vi "runStraight1Tote.vi"(11 "Distance In":dbl) -> ()   [LabVIEW 2015]
uses:
  Robot Global Data.vi
  <vilib>/addons/control/pid/NI_PID_pid.lvlib
  <vilib>/addons/control/pid/pid.llb/PID (DBL).vi
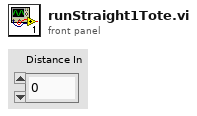
[diagram p1: front panel]
types:
  T1 = typedef "WPI_GyroDevRef.ctl" = cluster{"DevStatus":errorcluster, "Analog Channel":T2, "Offset":dbl, "Gain (VoltsPerDegree/Second)":dbl, "Gyro Type":enum16{"Analog", "XRS450"}, "Handle":i32, "SPI Bus":T3, "Device Found":bool, "Sample Rate":dbl, "Calibrate On Open":bool}
  T2 = typedef "FPGA_AIChannel.ctl" = enum8{"AI 0", "AI 1", "AI 2", "AI 3", "AI MXP 0", "AI MXP 1", "AI MXP 2", "AI MXP 3", "Invalid"}
  T3 = typedef "spi_bus.ctl" = enum16{"SPI On-Board, CS0", "SPI On-Board, CS1", "SPI On-Board, CS2", "SPI On-Board, CS3", "SPI MXP", "Invalid"}
  T4 = typedef "WPI_EncoderDevRef.ctl" = cluster{"DevStatus":errorcluster, "EncoderIndex":T5, "CounterIndex":T6, "DistancePerCount":dbl, "Decoding Type":T7}
  T5 = typedef "FPGA_EncoderIdx.ctl" = enum8{"Enc 0", "Enc 1", "Enc 2", "Enc 3", "Enc 4", "Enc 5", "Enc 6", "Enc 7", "Invalid"}
  T6 = typedef "FPGA_CounterCtrSystemIndex.ctl" = enum8{"Ctr 0", "Ctr 1", "Ctr 2", "Ctr 3", "Ctr 4", "Ctr 5", "Ctr 6", "Ctr 7", "Invalid"}
  T7 = typedef "WPI_EncoderType.ctl" = enum16{"1x", "2x", "4x"}
  T8 = cluster{"proportional gain (Kc)":dbl, "integral time (Ti, min)":dbl, "derivative time (Td, min)":dbl}
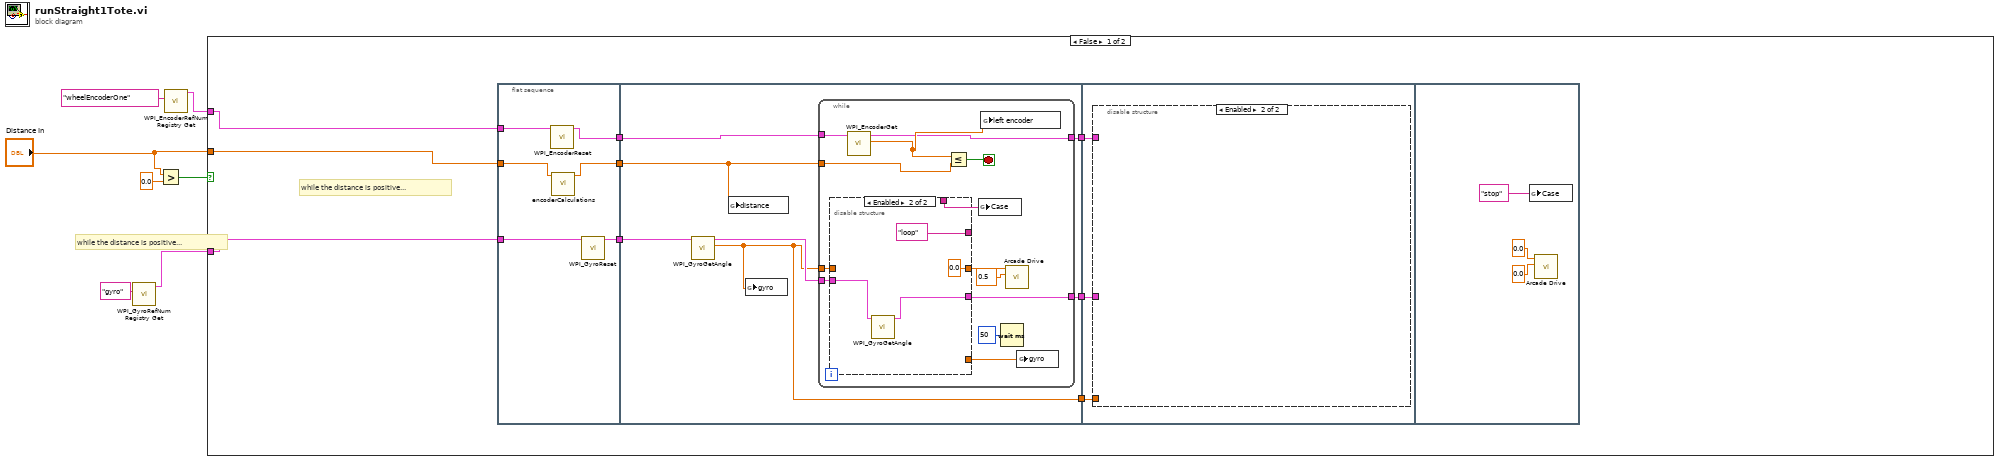
[diagram p0: block diagram]
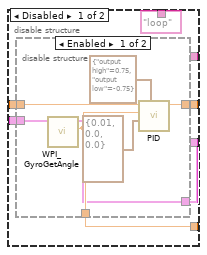
[diagram p2: hidden frame]
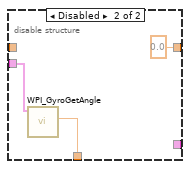
[diagram p3: hidden frame]
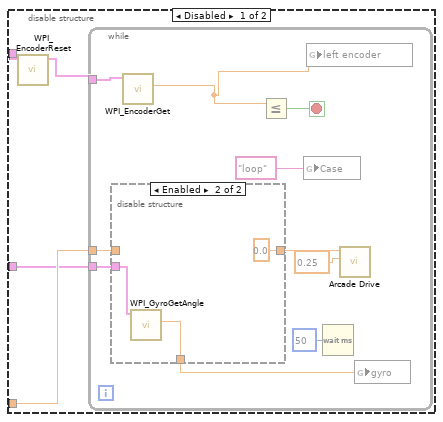
[diagram p4: hidden frame]
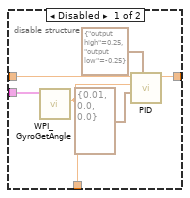
[diagram p5: hidden frame]
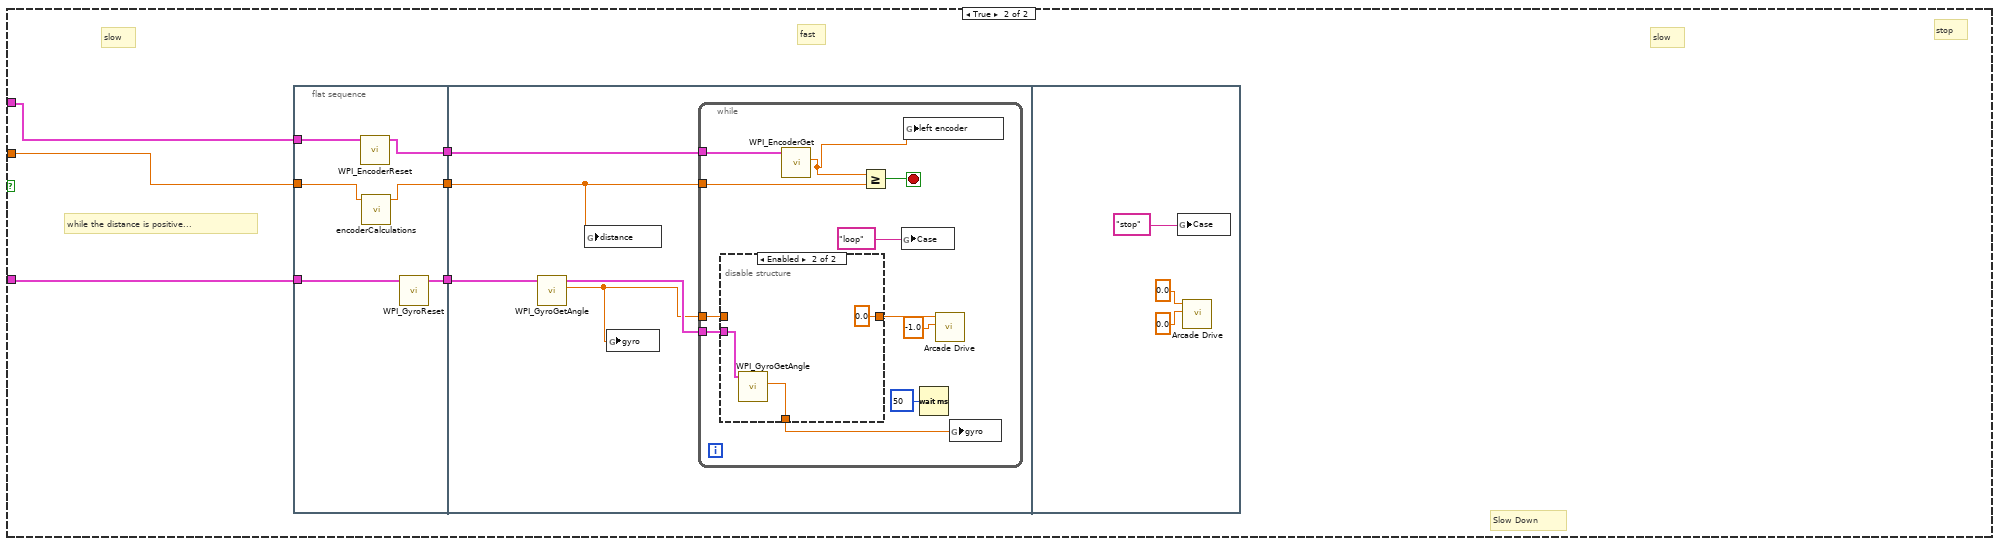
[diagram p6: hidden frame]
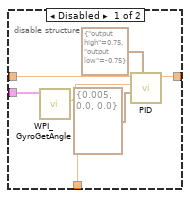
[diagram p7: hidden frame]
diagram:
  # "while the distance is positive..."
  n1 = call <vilib>:"WPI_GyroRefNum Registry Get.vi"("refnum name"="gyro") -> ("GyroDevRef"=w1:T1)  [unwired: 9 in, 1 out]
  n2 = Greater?(x="Distance In", y=0.0) -> (0:w6:bool)
  n3 = call <vilib>:"WPI_EncoderRefNum Registry Get.vi"("refnum name"="wheelEncoderOne") -> ("EncoderDevRef"=w3:T4)  [unwired: 9 in, 1 out]
  n4 = case shown="False" w6 {
    tunnel: "Distance In" -> [w12 w95]
    tunnel: w3 -> [w13 w93]
    tunnel: w1 -> [w11 w94]
    frame False {
      # "while the distance is positive..."
      n5 = flat-sequence {
        tunnel: w12 -> [w21]
        tunnel: [w20] -> w16
        tunnel: [w22] -> w15
        tunnel: w11 -> [w19]
        tunnel: w13 -> [w18]
        tunnel: [w17] -> w14
        tunnel: w16 -> [w27]
        tunnel: w15 -> [w28]
        tunnel: w14 -> [w26]
        tunnel: [w25] -> w10
        tunnel: [w24] -> w9
        tunnel: [w23] -> w8
        tunnel: w10 -> [w65]
        tunnel: w9 -> [w64]
        tunnel: w8 -> [w63]
        frame #0 {
          n6 = call <vilib>:"WPI_EncoderReset.vi"("EncoderDevRef"=w18) -> ("EncoderDevRef"=w17:T4)  [unwired: 9 in, 1 out]
          n7 = call "encoderCalculations.vi"("Left Distance In"=w21) -> ("Left Ticks"=w20:dbl)  [unwired: 9 in, 1 out]
          n8 = call <vilib>:"WPI_GyroReset.vi"("GyroDevRef"=w19) -> ("GyroDevRef"=w22:T1)  [unwired: 9 in, 1 out]
        }
        frame #1 {
          n9 = call <vilib>:"WPI_GyroGetAngle.vi"("GyroDevRef"=w28) -> ("Angle"=w24:dbl, "GyroDevRef"=w29:T1)  [unwired: 6 in, 3 out]
          n10 = global write "Robot Global Data.vi" "distance"(w27) -> ()
          n11 = global write "Robot Global Data.vi" "gyro"(w24) -> ()
          n12 = while {
            tunnel: w27 -> [w30]
            tunnel: w24 -> [w41]
            tunnel: w29 -> [w40]
            tunnel: w26 -> [w33]
            tunnel: [w32] -> w25
            tunnel: [w31] -> w23
            stop <- w42 stop-if-true
            n13 = disable-structure shown="Enabled" {
              disable-tunnel: w41 -> [w48 _]
              disable-tunnel: w40 -> [w47 w60]
              disable-tunnel: [w46 0.0 ("x")] -> w39
              disable-tunnel: ["loop" _] -> w37
              disable-tunnel: [w44 _] -> w34
              disable-tunnel: [w43 w61] -> w31
              disable-tunnel: [_ "loop"] -> _
              frame Disabled {
                n14 = disable-structure shown="Enabled" {
                  disable-tunnel: w48 -> [w53 _]
                  disable-tunnel: w47 -> [w52 w56]
                  disable-tunnel: [w51 0.0 ("x")] -> w46
                  disable-tunnel: [w50 w57] -> w44
                  disable-tunnel: [w49 _] -> w43
                  frame Enabled {
                    n15 = call <vilib>:"WPI_GyroGetAngle.vi"("GyroDevRef"=w52) -> ("Angle"=w50:dbl, "GyroDevRef"=w49:T1)  [unwired: 6 in, 3 out]
                    n16 = call-poly <vilib>:"PID.vi"("output range"=cluster{"output high":dbl, "output low":dbl} {"output high"=0.75, "output low"=-0.75}, "PID gains"=T8 {"proportional gain (Kc)"=0.01, "integral time (Ti, min)"=0.0, "derivative time (Td, min)"=0.0}, "process variable"=w50, "setpoint"=w53) -> ("output"=w51:dbl)  [unwired: 6 in, 1 out]
                  }
                  frame Disabled {
                    n17 = call <vilib>:"WPI_GyroGetAngle.vi"("GyroDevRef"=w56) -> ("Angle"=w57:dbl)  [unwired: 6 in, 4 out]
                  }
                }
              }
              frame Enabled {
                n18 = call <vilib>:"WPI_GyroGetAngle.vi"("GyroDevRef"=w60) -> ("GyroDevRef"=w61:T1)  [unwired: 6 in, 4 out]
              }
            }
            n19 = call <vilib>:"WPI_EncoderGet.vi"("EncoderDevRef"=w33) -> ("Distance"=w35:dbl, "EncoderDevRef"=w32:T4)  [unwired: 5 in, 4 out]
            n20 = Less Or Equal?(x=w35, y=w30) -> (x <= y?=w42:bool)
            n21 = global write "Robot Global Data.vi" "Case"(w37) -> ()
            n22 = global write "Robot Global Data.vi" "left encoder"(w35) -> ()
            n23 = Wait (ms)(milliseconds to wait=u32 50) -> ()  [unwired: 1 out]
            n24 = call "Arcade Drive.vi"("y"=0.5, "x"=w39) -> ()  [unwired: 10 in]
            n25 = global write "Robot Global Data.vi" "gyro"(w34) -> ()
          }
        }
        frame #2 {
          n26 = disable-structure shown="Enabled" {
            disable-tunnel: w65 -> [w69 _]
            disable-tunnel: w64 -> [w67 _]
            disable-tunnel: w63 -> [w66 _]
            frame Disabled {
              n27 = call <vilib>:"WPI_EncoderReset.vi"("EncoderDevRef"=w69) -> ("EncoderDevRef"=w68:T4)  [unwired: 9 in, 1 out]
              n28 = while {
                tunnel: w67 -> [w78]
                tunnel: w66 -> [w77]
                tunnel: w68 -> [w70]
                stop <- w79 stop-if-true
                n29 = disable-structure shown="Enabled" {
                  disable-tunnel: w78 -> [w83 _]
                  disable-tunnel: w77 -> [w82 w86]
                  disable-tunnel: [w81 0.0 ("x")] -> w76
                  disable-tunnel: [w80 w87] -> w71
                  frame Disabled {
                    n30 = call <vilib>:"WPI_GyroGetAngle.vi"("GyroDevRef"=w82) -> ("Angle"=w80:dbl)  [unwired: 6 in, 4 out]
                    n31 = call-poly <vilib>:"PID.vi"("output range"=cluster{"output high":dbl, "output low":dbl} {"output high"=0.25, "output low"=-0.25}, "PID gains"=T8 {"proportional gain (Kc)"=0.01, "integral time (Ti, min)"=0.0, "derivative time (Td, min)"=0.0}, "process variable"=w80, "setpoint"=w83) -> ("output"=w81:dbl)  [unwired: 6 in, 1 out]
                  }
                  frame Enabled {
                    n32 = call <vilib>:"WPI_GyroGetAngle.vi"("GyroDevRef"=w86) -> ("Angle"=w87:dbl)  [unwired: 6 in, 4 out]
                  }
                }
                n33 = call <vilib>:"WPI_EncoderGet.vi"("EncoderDevRef"=w70) -> ("Distance"=w72:dbl)  [unwired: 5 in, 5 out]
                n34 = Less Or Equal?(x=w72) -> (x <= y?=w79:bool)  [unwired: 1 in]
                n35 = global write "Robot Global Data.vi" "Case"("loop") -> ()
                n36 = global write "Robot Global Data.vi" "left encoder"(w72) -> ()
                n37 = Wait (ms)(milliseconds to wait=u32 50) -> ()  [unwired: 1 out]
                n38 = call "Arcade Drive.vi"("y"=0.25, "x"=w76) -> ()  [unwired: 10 in]
                n39 = global write "Robot Global Data.vi" "gyro"(w71) -> ()
              }
            }
            frame Enabled {
            }
          }
        }
        frame #3 {
          n40 = global write "Robot Global Data.vi" "Case"("stop") -> ()
          n41 = call "Arcade Drive.vi"("y"=0.0, "x"=0.0) -> ()  [unwired: 10 in]
        }
      }
    }
    frame True {
      # "stop"
      # "slow"
      # "fast"
      # "slow"
      # "while the distance is positive..."
      # "Slow Down"
      n42 = flat-sequence {
        tunnel: w95 -> [w102]
        tunnel: [w101] -> w97
        tunnel: [w103] -> w96
        tunnel: w94 -> [w100]
        tunnel: w93 -> [w99]
        tunnel: [w98] -> w92
        tunnel: w97 -> [w105]
        tunnel: w96 -> [w106]
        tunnel: w92 -> [w104]
        frame #0 {
          n43 = call <vilib>:"WPI_EncoderReset.vi"("EncoderDevRef"=w99) -> ("EncoderDevRef"=w98:T4)  [unwired: 9 in, 1 out]
          n44 = call "encoderCalculations.vi"("Left Distance In"=w102) -> ("Left Ticks"=w101:dbl)  [unwired: 9 in, 1 out]
          n45 = call <vilib>:"WPI_GyroReset.vi"("GyroDevRef"=w100) -> ("GyroDevRef"=w103:T1)  [unwired: 9 in, 1 out]
        }
        frame #1 {
          n46 = call <vilib>:"WPI_GyroGetAngle.vi"("GyroDevRef"=w106) -> ("Angle"=w107:dbl, "GyroDevRef"=w108:T1)  [unwired: 6 in, 3 out]
          n47 = global write "Robot Global Data.vi" "distance"(w105) -> ()
          n48 = global write "Robot Global Data.vi" "gyro"(w107) -> ()
          n49 = while {
            tunnel: w105 -> [w119]
            tunnel: w107 -> [w117]
            tunnel: w108 -> [w116]
            tunnel: w104 -> [w109]
            stop <- w118 stop-if-true
            n50 = disable-structure shown="Enabled" {
              disable-tunnel: w117 -> [w123 _]
              disable-tunnel: w116 -> [w122 w126]
              disable-tunnel: [w121 0.0 ("x")] -> w115
              disable-tunnel: [w120 w127] -> w110
              frame Disabled {
                n51 = call <vilib>:"WPI_GyroGetAngle.vi"("GyroDevRef"=w122) -> ("Angle"=w120:dbl)  [unwired: 6 in, 4 out]
                n52 = call-poly <vilib>:"PID.vi"("output range"=cluster{"output high":dbl, "output low":dbl} {"output high"=0.75, "output low"=-0.75}, "PID gains"=T8 {"proportional gain (Kc)"=0.005, "integral time (Ti, min)"=0.0, "derivative time (Td, min)"=0.0}, "process variable"=w120, "setpoint"=w123) -> ("output"=w121:dbl)  [unwired: 6 in, 1 out]
              }
              frame Enabled {
                n53 = call <vilib>:"WPI_GyroGetAngle.vi"("GyroDevRef"=w126) -> ("Angle"=w127:dbl)  [unwired: 6 in, 4 out]
              }
            }
            n54 = call <vilib>:"WPI_EncoderGet.vi"("EncoderDevRef"=w109) -> ("Distance"=w111:dbl)  [unwired: 5 in, 5 out]
            n55 = Greater Or Equal?(x=w111, y=w119) -> (x >= y?=w118:bool)
            n56 = global write "Robot Global Data.vi" "Case"("loop") -> ()
            n57 = global write "Robot Global Data.vi" "left encoder"(w111) -> ()
            n58 = Wait (ms)(milliseconds to wait=u32 50) -> ()  [unwired: 1 out]
            n59 = call "Arcade Drive.vi"("y"=-1.0, "x"=w115) -> ()  [unwired: 10 in]
            n60 = global write "Robot Global Data.vi" "gyro"(w110) -> ()
          }
        }
        frame #2 {
          n61 = global write "Robot Global Data.vi" "Case"("stop") -> ()
          n62 = call "Arcade Drive.vi"("y"=0.0, "x"=0.0) -> ()  [unwired: 10 in]
        }
      }
    }
  }
